vi "Get Sequence State.vi"(8 "error in (no error)":errorcluster, 10 "Sequence Name":string, 11 "Session Ref in":T2) -> (0 "error out":errorcluster, 1 "State":T1, 2 "Sequence Name out":string, 3 "Session Ref out":T2)   [LabVIEW 2020, in "NI_VS Sequence Execution Interface.lvlib"]
doc: "Returns the execution state of a real-time sequence (Idle, Running, SingleStepping, Paused, Complete)."
uses:
  <vilib>/NI VeriStand/Execution/SequenceExecutionInterface/NI_VS Sequence Execution Interface.lvlib
  <vilib>/NI VeriStand/Execution/SequenceExecutionInterface/Stimulus Profile Session Ref.ctl
  NationalInstruments.VeriStand.ClientAPI
  <vilib>/NI VeriStand/Execution/SequenceExecutionInterface/Sequence Execution State.ctl
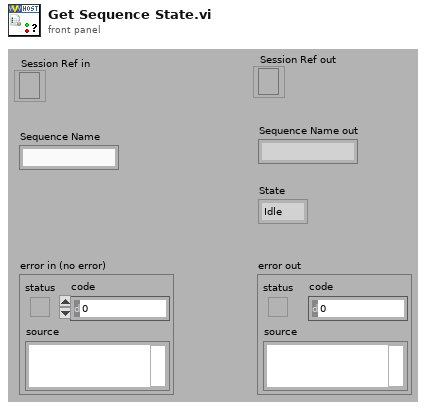
[diagram p1: front panel]
types:
  T1 = typedef "NI_VS Sequence Execution Interface.lvlib/Sequence Execution State.ctl" = enum16{"Idle", "Running", "SingleStepping", "Paused", "Stopped"}
  T2 = typedef "NI_VS Sequence Execution Interface.lvlib/Stimulus Profile Session Ref.ctl" = refnum<k24>
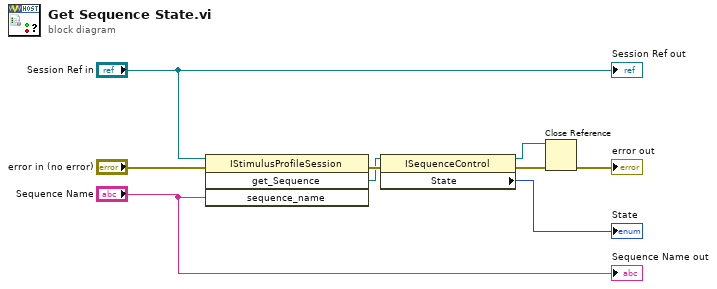
[diagram p0: block diagram]
diagram:
  n1 = invoke class="IStimulusProfileSession" method="get_Sequence"(reference="Session Ref in", error in="error in (no error)", "sequence_name"="Sequence Name") -> (error out=w6:errorcluster, "get_Sequence"=w5:refnum<k24>)  [unwired: 1 in, 2 out]
  n2 = property class="ISequenceControl"(reference=w5, error in=w6) -> (reference out=w4:refnum<k24>, error out=w3:errorcluster, "State"=→"State":i32)
  n3 = Close Reference(reference=w4, error in (no error)=w3) -> (error out=→"error out":errorcluster)
  "Session Ref out" <- "Session Ref in"
  "Sequence Name out" <- "Sequence Name"
